vi "fpga_Channel Index.vi"(8 "input valid? (T)":bool=TRUE, 11 "number of channels":T1=1 items=["1"=1, "2"=2, "3"=3, "4"=4, "5"=5, "6"=6, "7"=7, "8"=8, "9"=9, "10"=10, "11"=11, "12"=12, "13"=13, "14"=14, "15"=15, "16"=16]) -> (3 "channel index":u8)   [LabVIEW 2012, in "NI_EP_Protection_FPGA.lvlib"]
uses:
  <vilib>/addons/Electrical Power/PQ/Resampling/FPGA/subVIs/fpga_NofCH.ctl
  <vilib>/rvi/FXPMathLib/basic elements/FxpAddSub/XNode/nifxpmath_AddSub.xnode
  <vilib>/addons/Electrical Power/Protection/NI_EP_Protection_FPGA.lvlib
  <vilib>/rvi/FXPMathLib/sim/FxpSim.dll
  <vilib>/addons/Electrical Power/PQ/Resampling/NI_EP_Resample_FPGA.lvlib
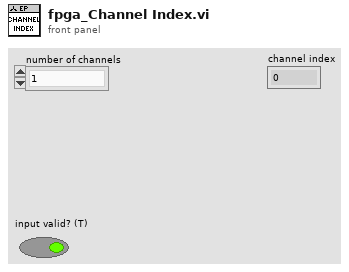
[diagram p1: front panel]
types:
  T1 = typedef "NI_EP_Resample_FPGA.lvlib/fpga_NofCH.ctl" = u8
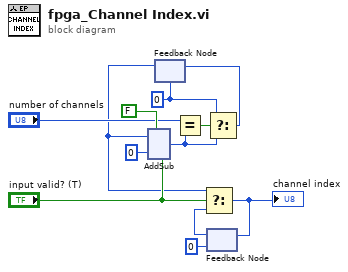
[diagram p0: block diagram]
diagram:
  w8 = u8 0 ("s")
  n1 = feedback #1(w8) -> (w1:u8)
  n2 = xnode "AddSub"("x"=w1, "y"=u8 0, "carry-in"="input valid? (T)", "use zero instead of x"=FALSE) -> ("s"=w6:u8)  [unwired: 1 out]
  n3 = Equal?(x="number of channels", y=w6) -> (x = y?=w9:bool)
  n4 = feedback #2(u8 0) -> (w11:u8)
  n5 = Select(t=w1, s="input valid? (T)", f=w11) -> (s? t:f=w12:u8)
  "channel index" <- w12
  n6 = feedback-in #2(w12) -> ()
  n7 = Select(t=w8, s=w9, f=w6) -> (s? t:f=w4:u8)
  n8 = feedback-in #1(w4) -> ()
